vi "test core.vi"(8 "error in (no error)":errorcluster, 11 "Network Actor in":refnum<class "Network Actor.lvclass">) -> (0 "error out":errorcluster)   [LabVIEW 2014, in "Network Actor Library.lvlib" / "Network Actor.lvclass"]
uses:
  Network Actor.lvclass
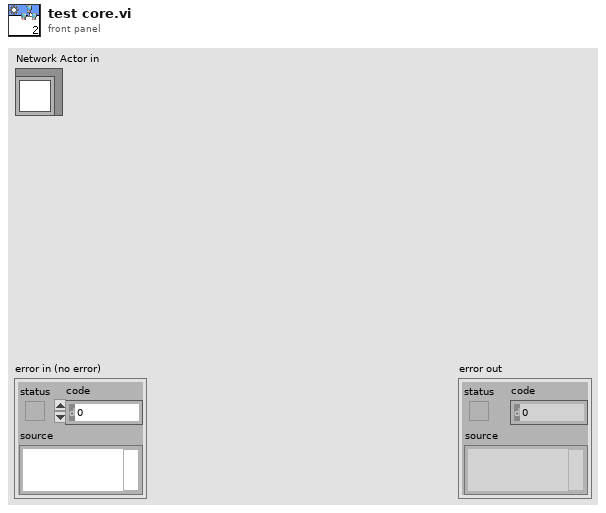
[diagram p1: front panel]
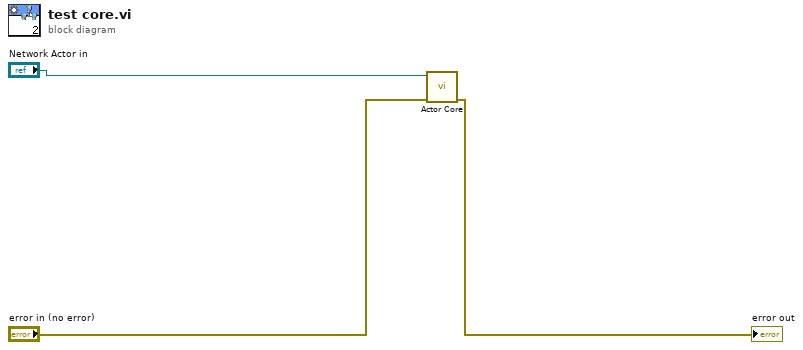
[diagram p0: block diagram]
diagram:
  n1 = call-dynamic "Actor Core.vi"("error in"="error in (no error)", "Network Actor in"="Network Actor in") -> ("error out"=→"error out":errorcluster)  [unwired: 8 in, 1 out]
